vi "Copy Image To Picture (16-bit).vi"(8 "error in (no error)":errorcluster, 11 "image_ptr":i64) -> (0 "error out":errorcluster, 3 "Image (16-bit)":T1)   [LabVIEW 2020, in "G-Image.lvlib"]
doc: "Read the image data from the pointer into LabVIEW, then free the memory. The image is returned as a LabVIEW picture."
uses:
  G-Image.lvlib
  Image IO/Controls/Image 16-bit.ctl
  66916a40-e4f8-49d9-be15-b4efa5ca52e6.vi
  d5bb44f2-3ba0-4077-8bde-e7ea6f1f76c1.vi
  b9f83168-43ce-4319-9b2d-e8672f8e3a99.vi
  <vilib>/Utility/error.llb/Error Cluster From Error Code.vi
  lib/g_image_32.dll
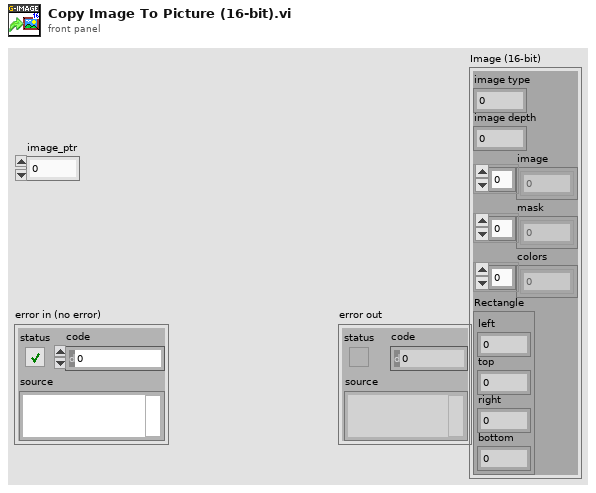
[diagram p1: front panel]
types:
  T1 = typedef "G-Image.lvlib/Image 16-bit.ctl" = cluster{"image type":i32, "image depth":i32, "image":u16[], "mask":u8[], "colors":u32[], "Rectangle":cluster{"left":i16, "top":i16, "right":i16, "bottom":i16}}
  T2 = cluster{"data":i32, "colors":i32, "delays":i32, "data_size":i32, "color_size":i32, "width":i32, "height":i32, "channels":i32, "bits_per_channel":i32, "layers":i32}
  T3 = cluster{"data":i64, "colors":i64, "delays":i64, "data_size":i32, "color_size":i32, "width":i32, "height":i32, "channels":i32, "bits_per_channel":i32, "layers":i32}
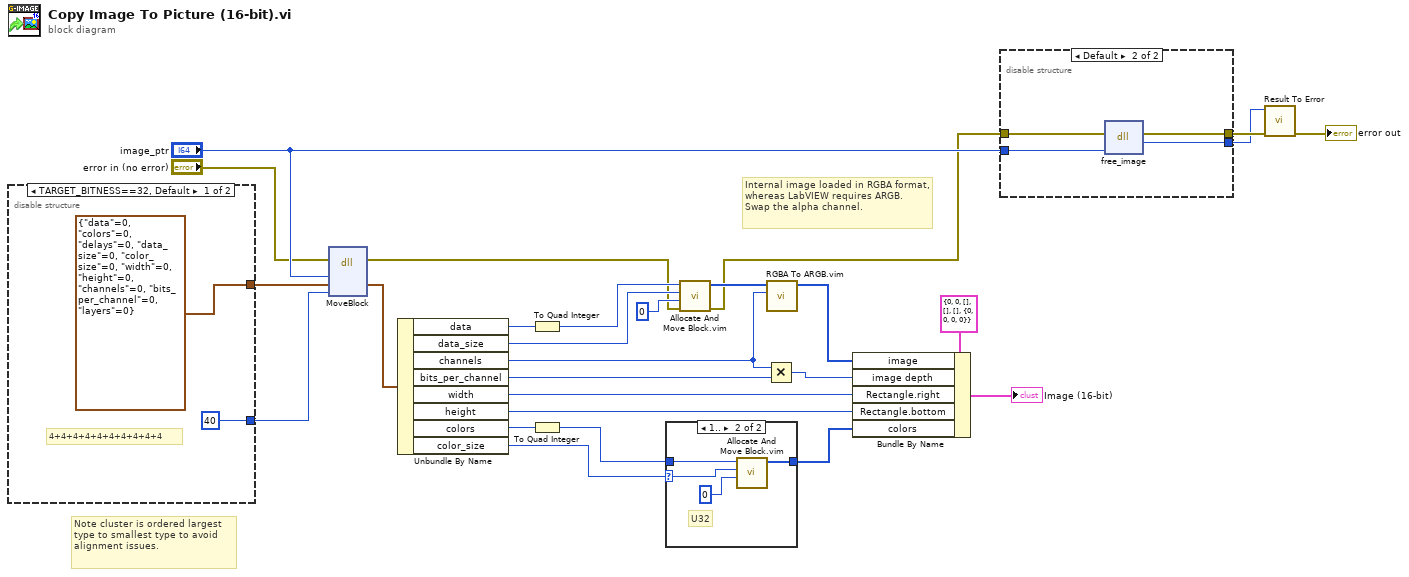
[diagram p0: block diagram]
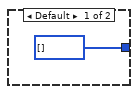
[diagram p2: hidden frame]
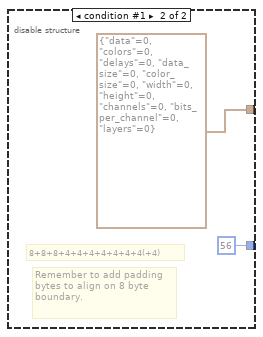
[diagram p3: hidden frame]
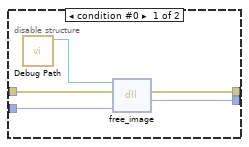
[diagram p4: hidden frame]
diagram:
  # "Internal image loaded in RGBA format, whereas LabVIEW requires ARGB. Swap the alpha channel."
  # "Note cluster is ordered largest type to smallest type to avoid alignment issues."
  n1 = disable-structure shown="TARGET_BITNESS==32, Default" {
    disable-tunnel: [T2 {"data"=0, "colors"=0, "delays"=0, "data_size"=0, "color_size"=0, "width"=0, "height"=0, "channels"=0, "bits_per_channel"=0, "layers"=0} T3 {"data"=0, "colors"=0, "delays"=0, "data_size"=0, "color_size"=0, "width"=0, "height"=0, "channels"=0, "bits_per_channel"=0, "layers"=0}] -> w21
    disable-tunnel: [40 ("x") 56 ("x")] -> w23
    frame condition #0 (active) {
      # "4+4+4+4+4+4+4+4+4+4"
    }
    frame condition #1 {
      # "Remember to add padding bytes to align on 8 byte boundary."
      # "8+8+8+4+4+4+4+4+4+4(+4)"
    }
  }
  n2 = dll-call lib="LabVIEW" fn="MoveBlock"(error in="error in (no error)", "Address (Pointer)"="image_ptr", "Destination"=w21, "Size"=w23) -> (error out=w6:errorcluster, "Destination"=w22:T2)  [unwired: 5 in, 1 out]
  n3 = Unbundle By Name(w22) -> ("data"=w10:i32, "data_size"=w11:i32, "channels"=w1:i32, "bits_per_channel"=w4:i32, "width"=w20:i32, "height"=w19:i32, "colors"=w14:i32, "color_size"=w13:i32)
  n4 = To Quad Integer(1:w10) -> (0:w7:i64)
  n5 = To Quad Integer(1:w14) -> (0:w12:i64)
  n6 = case shown="1.." w13 {
    selector: w13 -> [_ w36]
    tunnel: [u32[] [] ("Destination") w34] -> w15
    tunnel: w12 -> [_ w33]
    frame Default {
    }
    frame 1.. {
      # "U32"
      n7 = call "Allocate And Move Block.vim"("Type"=u32 0 ("element"), "Count"=w36, "Address"=w33) -> ("Data"=w34:u32[])  [unwired: 7 in, 1 out]
    }
  }
  n8 = call "Allocate And Move Block.vim"("error in (no error)"=w6, "Type"=u16 0 ("element"), "Count"=w11, "Address"=w7) -> ("error out"=w5:errorcluster, "Data"=w8:u16[])  [unwired: 6 in]
  n9 = Multiply(x=w1, y=w4) -> (x*y=w3:i32)
  n10 = call "RGBA To ARGB.vim"("Channels"=w1, "RGBA"=w8) -> ("ARGB"=w17:u16[])  [unwired: 9 in]
  n11 = Bundle By Name(cluster=T1 {"image type"=0, "image depth"=0, "image"=[], "mask"=[], "colors"=[], "Rectangle"={"left"=0, "top"=0, "right"=0, "bottom"=0}} ("Pixmap"), "image"=w17, "image depth"=w3, "Rectangle.right"=w20, "Rectangle.bottom"=w19, "colors"=w15) -> (→"Image (16-bit)":T1)
  n12 = disable-structure shown="Default" {
    disable-tunnel: w5 -> [w40 w45]
    disable-tunnel: [w39 w44] -> w25
    disable-tunnel: [w38 w43] -> w24
    disable-tunnel: "image_ptr" -> [w37 w42]
    frame condition #0 {
      n13 = call "Debug Path.vi"() -> ("Debug Path"=w41:path)  [unwired: 11 in]
      n14 = dll-call lib="?" fn="free_image"(path in=w41, error in=w40, "image_ptr"=w37) -> (error out=w39:errorcluster, "result"=w38:i32)  [unwired: 2 in, 1 out]
    }
    frame condition #1 (active) {
      n15 = dll-call lib="C:/github/dataflowg/g-image/src/LabVIEW/G-Image/lib/g_image_*.*" fn="free_image"(error in=w45, "image_ptr"=w42) -> (error out=w44:errorcluster, "result"=w43:i32)  [unwired: 3 in, 1 out]
    }
  }
  n16 = call "Result To Error.vi"("error in (no error)"=w25, "Result Code"=w24) -> ("error out"=→"error out":errorcluster)  [unwired: 9 in]
